vi "CheckStr.vi"(1 "String":string) -> (0 "s? t:f":string)   [LabVIEW 2017]
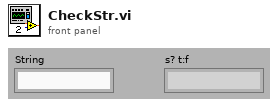
[diagram p1: front panel]
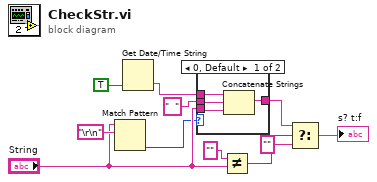
[diagram p0: block diagram]
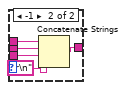
[diagram p2: hidden frame]
diagram:
  n1 = Match Pattern(string="String", regular expression="\r\n") -> (offset past match=w1:i32)  [unwired: 1 in, 3 out]
  n2 = Get Date/Time String(want seconds? (F)=TRUE) -> (time string=w8:string)  [unwired: 2 in, 1 out]
  n3 = case shown="0, Default" w1 {
    tunnel: "  " ("string") -> [w14 w20]
    tunnel: w8 -> [w15 w19]
    tunnel: [w12 w18] -> w7
    tunnel: "String" -> [w13 w17]
    frame 0, Default {
      n4 = Concatenate Strings(w15, w14, w13) -> (w12:string)
    }
    frame -1 {
      n5 = Concatenate Strings(w19, w20, w17, "\r\n") -> (w18:string)
    }
  }
  n6 = Not Equal?(x="", y="String") -> (x != y?=w6:bool)
  n7 = Select(t=w7, s=w6, f="") -> (s? t:f=→"s? t:f":string)
